vi "Write Harmonic.vi"(8 "error in (no error)":errorcluster, 10 "Harmonic":i8, 11 "Harmonics_CHP in":refnum<class "RxBN_CHP.lvclass">=refnum) -> (0 "error out":errorcluster, 3 "Harmonics_CHP out":refnum<class "RxBN_CHP.lvclass">)   [LabVIEW 2016]
uses:
  RxBN_CHP.lvclass
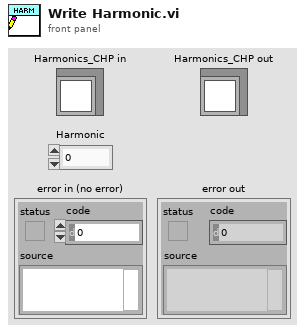
[diagram p1: front panel]
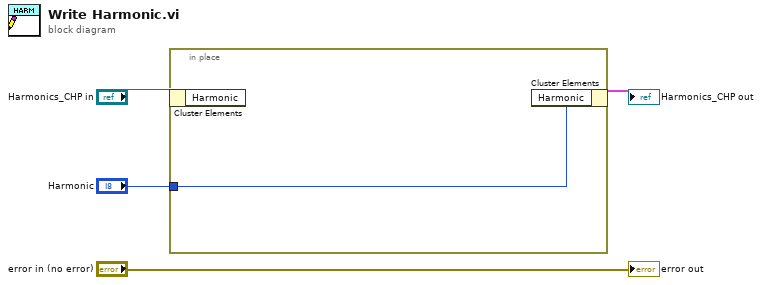
[diagram p0: block diagram]
diagram:
  n1 = in-place {
    in-place-border: "Harmonic" -> [w5]
    n2 = in-place-cluster #1("Harmonics_CHP in") -> ()  [unwired: 1 out]
    n3 = in-place-cluster #1("Harmonic"=w5) -> (→"Harmonics_CHP out":cluster{})
  }
  "error out" <- "error in (no error)"
